vi "timestamper.vi"(1 "seconds?":bool, 2 "ms?":bool) -> (0 "datetime output":string)   [LabVIEW 2010]
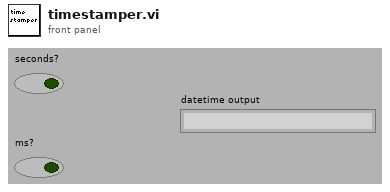
[diagram p1: front panel]
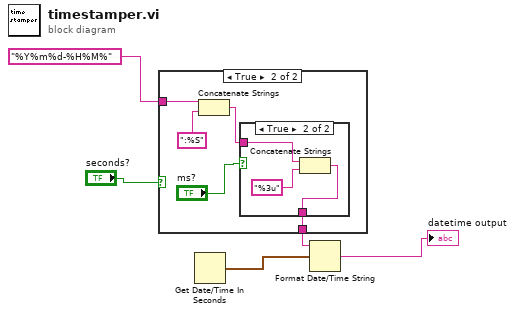
[diagram p0: block diagram]
diagram:
  n1 = case shown="True" "seconds?" {
    tunnel: "%Y%m%d-%H%M%" -> [w6 w10]
    tunnel: [w6 w8] -> w2
    frame False {
    }
    frame True {
      n2 = Concatenate Strings(w10, ":%S") -> (w9:string)
      n3 = case shown="True" "ms?" {
        tunnel: w9 -> [w12 w15]
        tunnel: [w12 w14] -> w8
        frame False {
        }
        frame True {
          n4 = Concatenate Strings(w15, "%3u") -> (w14:string)
        }
      }
    }
  }
  n5 = Get Date/Time In Seconds() -> (seconds since 1Jan1904=w5:timestamp)
  n6 = Format Date/Time String(time format string (%c)=w2, seconds (now)=w5) -> (date/time string=→"datetime output":string)  [unwired: 1 in]
